vi "DrawRobot.vi"(8 "error in (no error)":errorcluster, 10 "RobotPosition (m and rad)":cluster{"X":dbl, "Y":dbl, "Angle":dbl}, 11 "picture":picture) -> (0 "error out":errorcluster, 3 "new picture":picture)   [LabVIEW 2009, in "Host.lvlib" / "Draw.lvlib"]
uses:
  Draw.lvlib
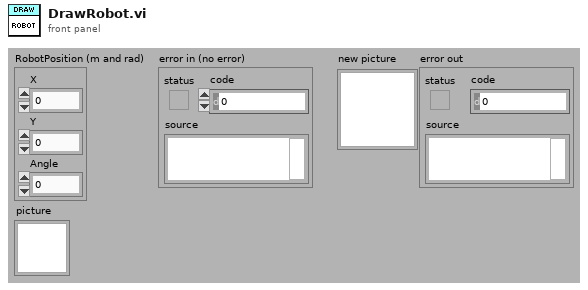
[diagram p1: front panel]
types:
  T1 = cluster{"Width":u16, "Style":enum32{"Solid", "Dash", "Dot", "DashDot", "DashDotDot"}}
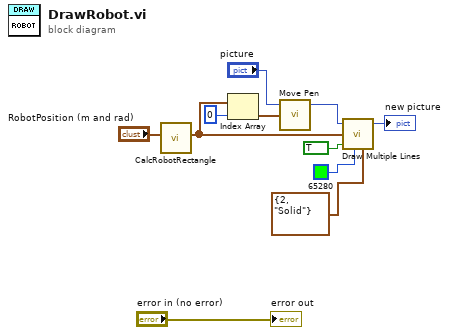
[diagram p0: block diagram]
diagram:
  n1 = call "CalcRobotRectangle.vi"("Position (m and rad)"="RobotPosition (m and rad)") -> ("line endpoints"=w4:cluster{"x":i16, "y":i16}[])  [unwired: 10 in]
  n2 = Index Array(array=w4, index=0) -> (element=w2:cluster{"x":i16, "y":i16})
  n3 = call <vilib>:"Move Pen.vi"("new position"=w2, "picture"="picture") -> ("new picture"=w11:picture)  [unwired: 3 in]
  n4 = call <vilib>:"Draw Multiple Lines.vi"("picture"=w11, "line endpoints"=w4, "fill?(F)"=TRUE, "color(black)"=u32 65280, "pen"=T1 {"Width"=2, "Style"=enum."Solid"}) -> ("new picture"=→"new picture":picture)  [unwired: 4 in]
  "error out" <- "error in (no error)"
